vi "TCP_CS장난감.vi"() -> ()   [LabVIEW 2018]
uses:
  <vilib>/LabVIEW Open Source Project/MQTT TCP Connection/MQTT_TCP/Connection/TCPConnection.lvclass
  C:/Program Files (x86)/National Instruments/LabVIEW 2018/vi.lib/LabVIEW Open Source Project/Connection/Connection/Connection.lvclass
  <vilib>/LabVIEW Open Source Project/Connection/Connection/Connection.lvclass
panel:
  out "문자열":string
  out "Comm OK":bool
  out "client connected":bool
  in  "전송":bool
  in  "보낸 문자열":string
  out "받은 문자열":string
  out "client session error":errorcluster
  in  "정지":bool
  out "server connected":bool
  out "listener error":errorcluster
  out "server session error":errorcluster
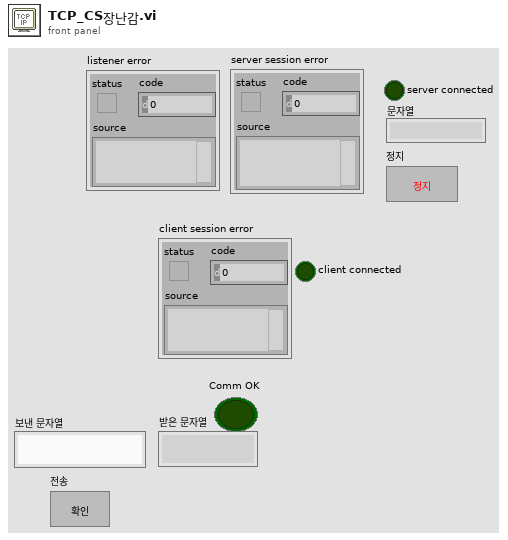
[diagram p1: front panel]
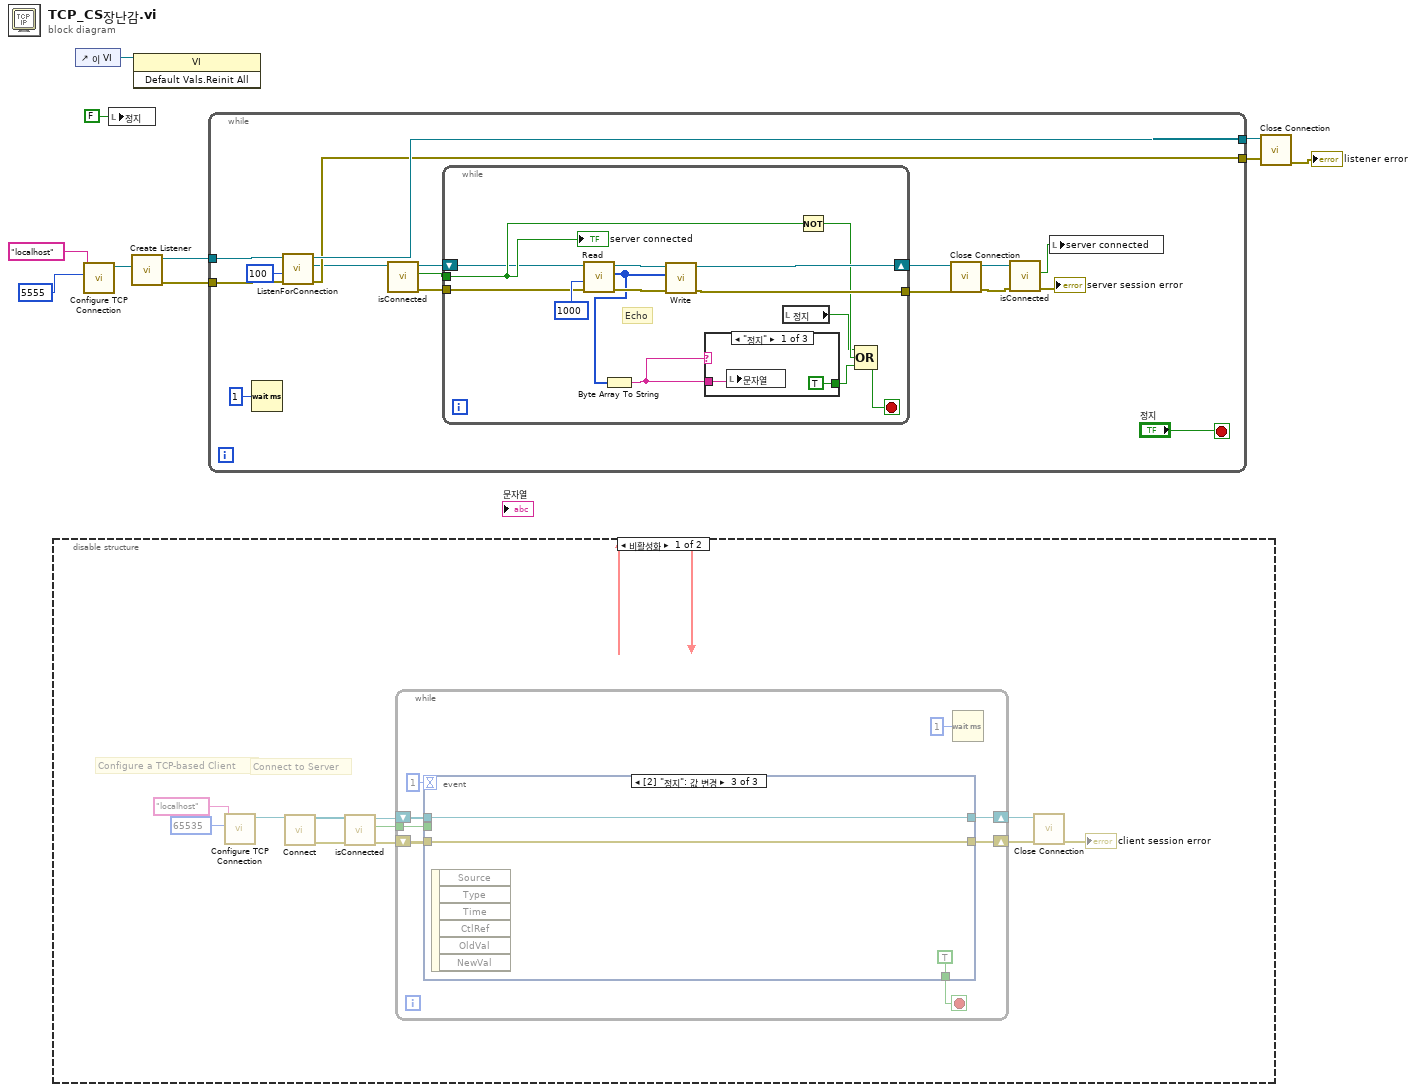
[diagram p0: block diagram]
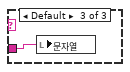
[diagram p3: hidden frame]
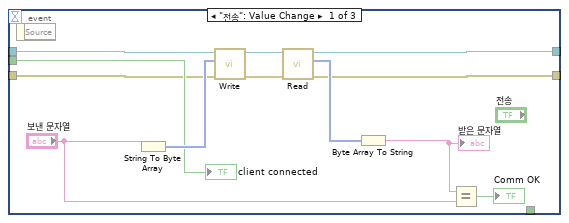
[diagram p4: hidden frame]
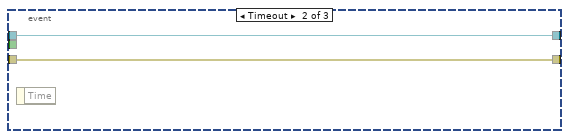
[diagram p5: hidden frame]
diagram:
  n1 = disable-structure shown="비활성화" {
    frame Disabled {
      # "Configure a TCP-based Client"
      # "Connect to Server"
      n2 = call <vilib>:"Configure TCP Connection.vi"("remote port (80)"=u16 65535, "address (localhost)"="localhost") -> ("TCPConnection"=w18:refnum<class "TCPConnection.lvclass">)  [unwired: 8 in, 1 out]
      n3 = call <vilib>:"Connect.vi"("Connection in"=w18) -> ("error out"=w14:errorcluster, "Connection out"=w12:refnum<class "TCPConnection.lvclass">)  [unwired: 9 in]
      n4 = call <vilib>:"isConnected.vi"("error in (no error)"=w14, "Connection in"=w12) -> ("error out"=w13:errorcluster, "connected"=w15:bool, "Connection out"=w11:refnum<class "TCPConnection.lvclass">)  [unwired: 7 in]
      n5 = while {
        tunnel: w15 -> [w27]
        shift-right: [w29] -> w20
        shift-left: w13 -> [w26]
        shift-right: [w28] -> w19
        shift-left: w11 -> [w25]
        stop <- w22 stop-if-true
        n6 = event shown="[2] \"정지\": 값 변경" {
          selector: _ -> [_ _ _]
          dyn-events: _ -> [_ _ _]
          timeout: 1 -> [_ _ _]
          tunnel: [w37 w42 w44] -> w29
          tunnel: [w36 w43 w45] -> w28
          tunnel: w27 -> [w34 _ _]
          tunnel: w26 -> [w33 w42 w44]
          tunnel: w25 -> [w32 w43 w45]
          tunnel: [_ _ TRUE ("정지")] -> w22
          event "전송": Value Change {
            n7 = event-data() -> ()  [unwired: 1 in, 1 out]
            n8 = String To Byte Array(string="보낸 문자열") -> (unsigned byte array=w39:u8[])
            n9 = call <vilib>:"Write.vi"("error in (no error)"=w33, "Bytes"=w39, "Connection in"=w32) -> ("error out"=w40:errorcluster, "Connection"=w41:refnum<class "TCPConnection.lvclass">)  [unwired: 7 in]
            n10 = call <vilib>:"Read.vi"("error in (no error)"=w40, "TCPConnection in"=w41) -> ("error out"=w37:errorcluster, "Bytes"=w38:u8[], "TCPConnection out"=w36:refnum<class "TCPConnection.lvclass">)  [unwired: 5 in, 2 out]
            n11 = Byte Array To String(unsigned byte array=w38) -> (string=w30:string)
            "받은 문자열" <- w30
            n12 = Equal?(x=w30, y="보낸 문자열") -> (x = y?=→"Comm OK":bool)
            "client connected" <- w34
          }
          event Timeout {
            n13 = event-data() -> ()  [unwired: 1 in, 1 out]
          }
          event "정지": Value Change {
            n14 = event-data() -> ()  [unwired: 1 in, 6 out]
          }
        }
        n15 = Wait (ms)(milliseconds to wait=u32 1 ("대기 시간 (ms)")) -> ()  [unwired: 1 out]
      }
      n16 = call <vilib>:"Close Connection.vi"("error in (no error)"=w20, "Connection in"=w19) -> ("error out"=→"client session error":errorcluster)  [unwired: 8 in, 1 out]
    }
    frame Enabled {
    }
  }
  n17 = control-ref of="이 VI"() -> (w5:refnum<vi>)
  n18 = call <vilib>:"Configure TCP Connection.vi"("remote port (80)"=u16 5555, "address (localhost)"="localhost") -> ("TCPConnection"=w8:refnum<class "TCPConnection.lvclass">)  [unwired: 8 in, 1 out]
  n19 = local write "정지"(FALSE ("정지")) -> ()
  n20 = call <vilib>:"Create Listener.vi"("Connection Configuration"=w8) -> ("error out"=w9:errorcluster, "Listener"=w10:refnum<class "TCPConnection.lvclass">)  [unwired: 9 in]
  n21 = invoke class="VI" method="Default Vals.Reinit All"(reference=w5) -> ()  [unwired: 2 in, 3 out]
  n22 = while {
    tunnel: w10 -> [w63]
    tunnel: w9 -> [w62]
    tunnel: [w58] -> w3
    tunnel: [w59] -> w2
    stop <- "정지" stop-if-true
    n23 = Wait (ms)(milliseconds to wait=u32 1 ("대기 시간 (ms)")) -> ()  [unwired: 1 out]
    n24 = call <vilib>:"ListenForConnection.vi"("error in (no error)"=w62, "timeout (2000 ms)"=100, "Listener"=w63) -> ("error out"=w58:errorcluster, "Connection"=w50:refnum<class "Connection.lvclass">, "Listener out"=w59:refnum<class "TCPConnection.lvclass">)  [unwired: 5 in, 1 out]
    n25 = call <vilib>:"isConnected.vi"("Connection in"=w50) -> ("error out"=w49:errorcluster, "connected"=w48:bool, "Connection out"=w47:refnum<class "Connection.lvclass">)  [unwired: 8 in]
    n26 = while {
      tunnel: [w73] -> w60
      shift-right: [w74] -> w61
      shift-left: w47 -> [w64]
      tunnel: w49 -> [w66]
      tunnel: w48 -> [w65]
      stop <- w68 stop-if-true
      # "Echo"
      n27 = call <vilib>:"Read.vi"("error in (no error)"=w66, "timeout (2000 ms)"=1000 ("bytes to read (100)"), "TCPConnection in"=w64) -> ("error out"=w75:errorcluster, "Bytes"=w72:u8[], "TCPConnection out"=w76:refnum<class "Connection.lvclass">)  [unwired: 4 in, 2 out]
      n28 = Byte Array To String(unsigned byte array=w72) -> (string=w71:string)
      n29 = call <vilib>:"Write.vi"("error in (no error)"=w75, "Bytes"=w72, "Connection in"=w76) -> ("error out"=w73:errorcluster, "Connection"=w74:refnum<class "Connection.lvclass">)  [unwired: 7 in]
      n30 = case shown="\"정지\"" w71 {
        tunnel: [TRUE _ _] -> w70
        tunnel: w71 -> [w78 _ w80]
        frame "정지" {
          n31 = local write "문자열"(w78) -> ()
        }
        frame "" {
        }
        frame Default {
          n32 = local write "문자열"(w80) -> ()
        }
      }
      n33 = local read "정지"() -> (w67:bool)
      n34 = Not(x=w65) -> (.not. x?=w69:bool)
      n35 = Compound Arithmetic op=OR ("복합 연산")(w67, w69, w70) -> (w68:bool)
      "server connected" <- w65
    }
    n36 = call <vilib>:"Close Connection.vi"("error in (no error)"=w60, "Connection in"=w61) -> ("error out"=w55:errorcluster, "No Connection"=w53:refnum<class "Connection.lvclass">)  [unwired: 8 in]
    n37 = call <vilib>:"isConnected.vi"("error in (no error)"=w55, "Connection in"=w53) -> ("error out"=→"server session error":errorcluster, "connected"=w52:bool)  [unwired: 7 in, 1 out]
    n38 = local write "server connected"(w52) -> ()
  }
  n39 = call <vilib>:"Close Connection.vi"("error in (no error)"=w3, "Connection in"=w2) -> ("error out"=→"listener error":errorcluster)  [unwired: 8 in, 1 out]
